vi "Read.vi"(8 "error in (no error)":errorcluster, 11 "Double Float.lvclass in":refnum<class "DAQmx-Bus_DBLType.lvclass">) -> (0 "error out":errorcluster, 2 "Value":T1, 3 "Double Float.lvclass out":refnum<class "DAQmx-Bus_DBLType.lvclass">)   [LabVIEW 2021, in "DAQmx-Bus_DBLType.lvclass"]
doc: "Abstract Data Classes 2.1.1.13\nTim Streeter - TSA\nCopyright (c) 2025, TSA"
uses:
  DAQmx-Bus_DBLType.lvclass
  <vilib>/TSA/Abstract Data Classes/Abs_Types/Double Float/Support/Type.ctl
  DAQmx-Bus_DBLType.lvclass/DAQmx-Bus_DBLType.ctl
  <vilib>/TSA/Abstract Data Classes/Abs_Types/Double Float/Abs_Double Float.lvclass
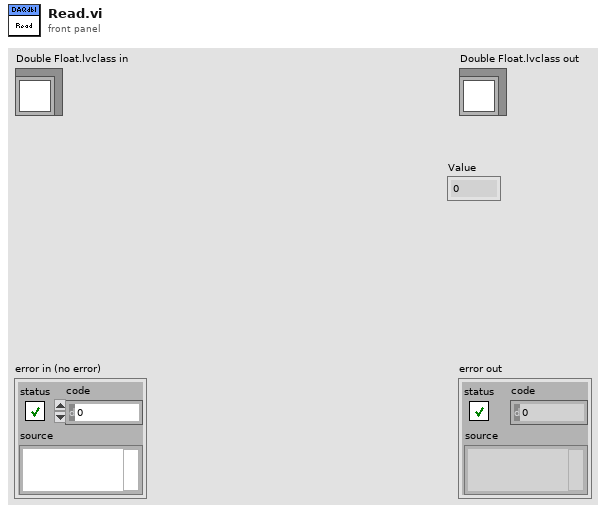
[diagram p1: front panel]
types:
  T1 = typedef "Abs_Double Float.lvclass/Type.ctl" = dbl
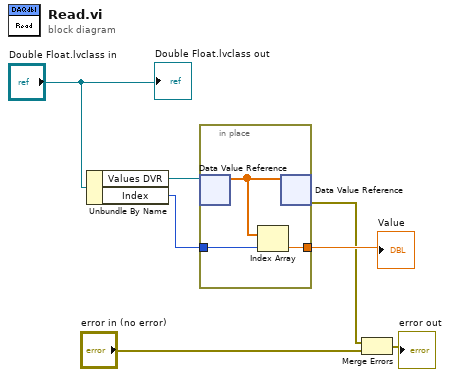
[diagram p0: block diagram]
diagram:
  n1 = Unbundle By Name("Double Float.lvclass in") -> ("Values DVR"=w6:refnum<data-value>, "Index"=w5:i32)
  n2 = in-place {
    in-place-border: w5 -> [w9]
    in-place-border: [w8] -> w4
    n3 = in-place-dvr #1(w6) -> (w10:dbl[])  [unwired: 1 out]
    n4 = Index Array(array=w10, index=w9) -> (element=w8:dbl)
    n5 = in-place-dvr #1(w10) -> (w1:errorcluster)  [unwired: 1 out]
  }
  "Value" <- w4
  n6 = Merge Errors(w1, "error in (no error)") -> (→"error out":errorcluster)
  "Double Float.lvclass out" <- "Double Float.lvclass in"
